vi "VisitLVEnumType.vi"(8 "error in (no error)":errorcluster, 10 "LVEnumType":refnum<class "LVEnum.lvclass">, 11 "GetTypeAttributesVisitor in":refnum<class "GetTypeAttributesVisitor.lvclass">) -> (0 "error out":errorcluster, 3 "GetTypeAttributesVisitor out":refnum<class "GetTypeAttributesVisitor.lvclass">)   [LabVIEW 2020, in "Web Service Description.lvlib" / "GetTypeAttributesVisitor.lvclass"]
uses:
  <vilib>/AppBuilder/Engine/WebServiceDescription/GetTypeAttributesVisitor/GetTypeAttributesVisitor.lvclass
  <vilib>/AppBuilder/Engine/WebServiceDescription/LVDataTypes/LVEnum/LVEnum.lvclass
  e:/builds/penguin/labview/branches/2020/dev/dist/vi.lib/AppBuilder/Engine/WebServiceDescription/LVDataTypes/LVType/LVType.lvclass
  <vilib>/AppBuilder/Engine/WebServiceDescription/XMLGen/ValuePair.ctl
  <vilib>/AppBuilder/Engine/WebServiceDescription/GetTypeAttributesVisitor/GetTypeAttributesVisitor.lvclass/GetTypeAttributesVisitor.ctl
  <vilib>/AppBuilder/Engine/WebServiceDescription/LVDataTypes/LVType/LVType.lvclass
  <vilib>/AppBuilder/Engine/WebServiceDescription/XMLGen/XMLGen.lvlib
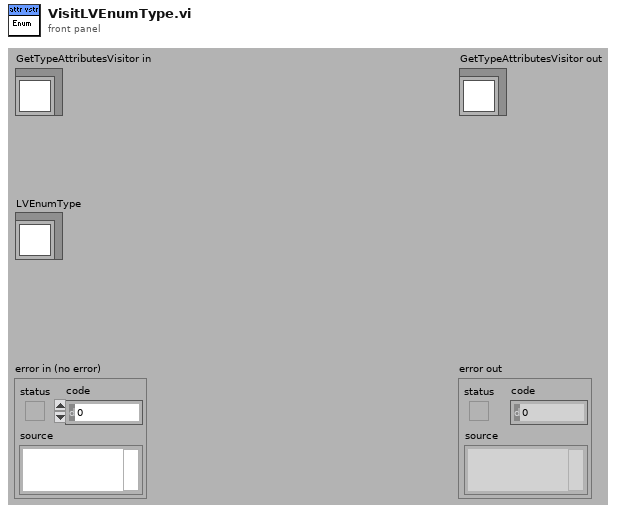
[diagram p1: front panel]
types:
  T1 = typedef "XMLGen.lvlib/ValuePair.ctl" = cluster{"Name":string, "Value":string}
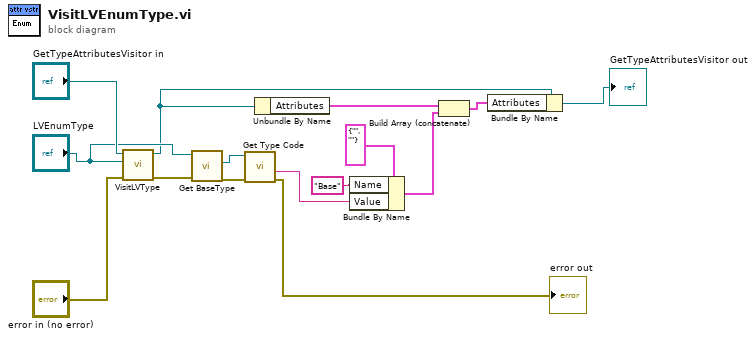
[diagram p0: block diagram]
diagram:
  n1 = call-dynamic "VisitLVType.vi"("error in (no error)"="error in (no error)", "LVType"="LVEnumType", "GetTypeAttributesVisitor in"="GetTypeAttributesVisitor in") -> ("error out"=w10:errorcluster, "GetTypeAttributesVisitor out"=w6:refnum<class "GetTypeAttributesVisitor.lvclass">)  [unwired: 7 out]
  n2 = call <vilib>:"Get BaseType.vi"("error in (no error)"=w10, "LVEnum.lvclass in"="LVEnumType") -> ("error out"=w12:errorcluster, "BaseType"=w13:refnum<class "LVType.lvclass">)  [unwired: 8 out]
  n3 = call <vilib>:"Get Type Code.vi"("error in (no error)"=w12, "LVType.lvclass in"=w13) -> ("error out"=→"error out":errorcluster, "TypeCodeString"=w7:string)  [unwired: 8 out]
  n4 = Unbundle By Name(w6) -> ("Attributes"=w5:T1[])
  n5 = Bundle By Name(cluster=T1 {"Name"="", "Value"=""} ("Attribute"), "Name"="Base", "Value"=w7) -> (w4:T1)
  n6 = Build Array (concatenate)(w5, w4) -> (w3:T1[])
  n7 = Bundle By Name(cluster=w6, "Attributes"=w3) -> (→"GetTypeAttributesVisitor out":refnum<class "GetTypeAttributesVisitor.lvclass">)
